vi "lsl create continuous resolver.vi"(8 "error in (no error)":errorcluster, 11 "forget_after":dbl) -> (0 "error out":errorcluster, 3 "function return":u32)   [LabVIEW 2016, in "Lab Streaming Layer.lvlib"]
doc: "extern LIBLSL_C_API lsl_continuous_resolver lsl_create_continuous_resolver(double forget_after);"
uses:
  Lab Streaming Layer.lvlib
  liblsl-LabVIEW-master/liblsl-LabVIEW-master/lsl.dll
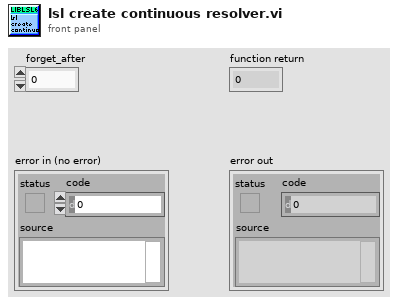
[diagram p1: front panel]
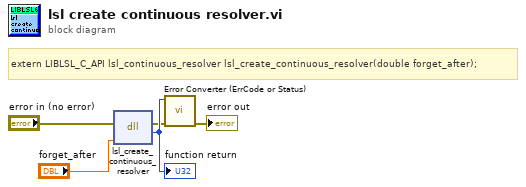
[diagram p0: block diagram]
diagram:
  # "extern LIBLSL_C_API lsl_continuous_resolver lsl_create_continuous_resolver(double forget_after);"
  n1 = dll-call lib="E:/LabStreamingLayer/liblsl-LabVIEW-master/liblsl-LabVIEW-master/lsl.dll" fn="lsl_create_continuous_resolver"(error in="error in (no error)", "forget_after"="forget_after") -> (error out=w2:errorcluster, "return type"=w5:u32)  [unwired: 3 in, 1 out]
  "function return" <- w5
  n2 = call "Error Converter (ErrCode or Status).vi"("error in (no error)"=w2, "error code"=w5) -> ("error out"=→"error out":errorcluster)  [unwired: 9 in]
